vi "05. Native MQTT Delegation.vi"() -> ()   [LabVIEW 2019]
uses:
  Actor/Request -- cluster.ctl
  <vilib>/LabVIEW Open Source Project/MQTT Control Packets/Control Packets/ControlPacket/ControlPacket.lvclass/ControlPacket.ctl
  d83398bf-d288-4447-9c56-1851baa950d7.vi
  <vilib>/LabVIEW Open Source Project/MQTT Control Packets/Control Packets/PUBLISH/PUBLISH.lvclass
  C:/Program Files (x86)/National Instruments/LabVIEW 2019/vi.lib/LabVIEW Open Source Project/MQTT Control Packets/Control Packets/ControlPacket/ControlPacket.lvclass
  <vilib>/JDP Science/JSONtext/JSON text to Variant.vi
  <vilib>/Utility/error.llb/Error Cluster From Error Code.vi
  <vilib>/JDP Science/JSONtext/LVClass Serializer/JSONtext LVClass Serializer.lvclass
  <vilib>/ErrorRing/Error Ring.xnode
  <vilib>/LabVIEW Open Source Project/MQTT Control Packets/Control Packets/ControlPacket/ControlPacket.lvclass
  <vilib>/JDP Science/JSONtext/JSONtext.lvlib
  <vilib>/ptbypt/NI_PtbyPt.lvlib
panel:
  in  "amplitude":dbl(slide)=2.0 scale=0.0..10.0
  out "<JSON>Response":string
  out "<JSON>":string caption="<JSON>Request"
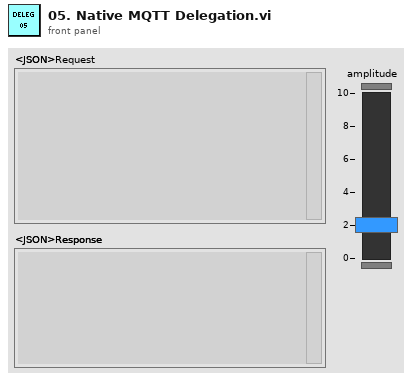
[diagram p1: front panel]
types:
  T1 = typedef "Actor Private Data.ctl" = cluster{"Client":refnum<class "Client.lvclass">, "QualifiedName":string, "EventReg":refnum<event-registration>, "Private Events":T2}
  T2 = typedef "Actor Private Events -- cluster.ctl" = cluster{"Stop":refnum<user-event>, "Subscribe":refnum<user-event>, "Unsubscribe":refnum<user-event>, "publish":refnum<user-event>}
  T3 = typedef "Request -- cluster.ctl" = cluster{"method":string, "<JSON>params":string, "id":string, "reply-topic":string}
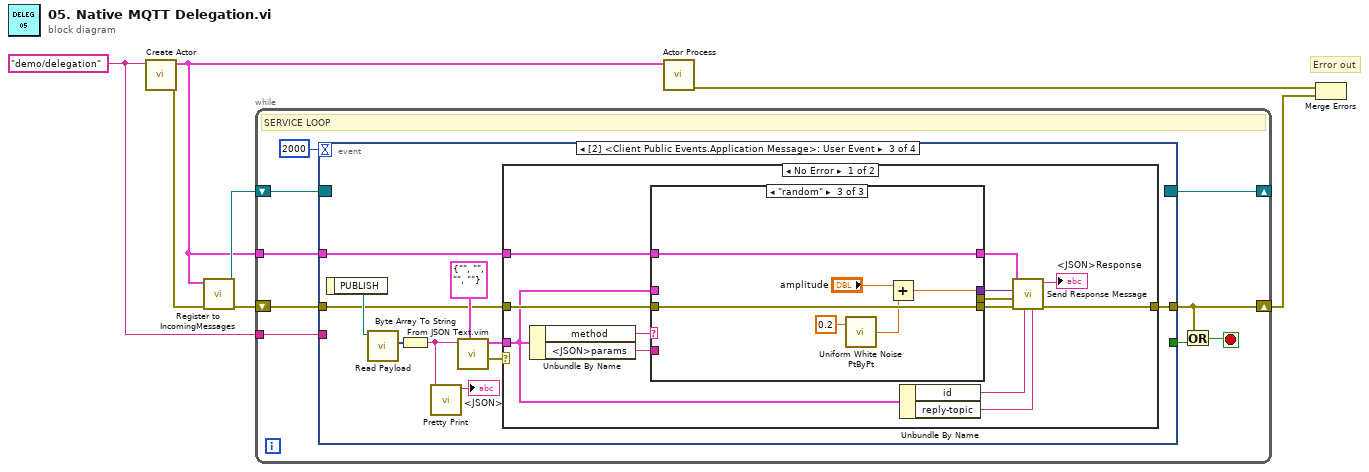
[diagram p0: block diagram]
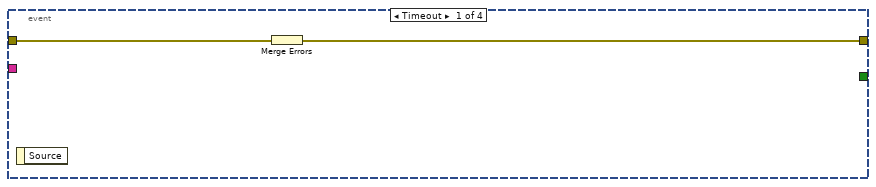
[diagram p2: hidden frame]
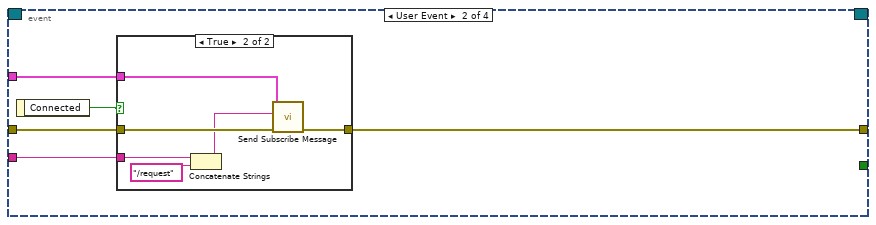
[diagram p3: hidden frame]
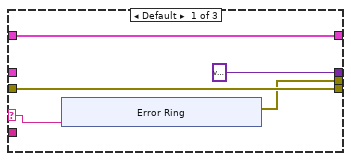
[diagram p5: hidden frame]
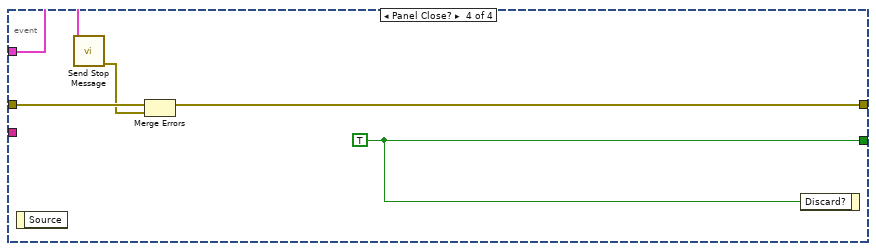
[diagram p8: hidden frame]
diagram:
  w2 = "demo/delegation" ("QualifiedName")
  # "Error out"
  n1 = call "Create Actor.vi"("QualifiedName"=w2) -> ("error out"=w6:errorcluster, "Actor Class"=w4:T1)  [unwired: 9 in]
  n2 = call "Register to IncomingMessages.vi"("error in"=w6, "Actor Class"=w4) -> ("error out"=w3:errorcluster, "Incoming Messages"=w5:refnum<event-registration>)  [unwired: 8 in]
  n3 = while {
    tunnel: w4 -> [w14]
    shift-right: [w11] -> _
    shift-left: w5 -> [w12]
    shift-right: [w9] -> w1
    shift-left: w3 -> [w10]
    tunnel: w2 -> [w8]
    stop <- w15 stop-if-true
    # "SERVICE LOOP"
    n4 = event shown="[2] <Client Public Events.Application Message>: User Event" {
      selector: w12 -> [_ _ _ _]
      dyn-events: [_ _ _ _] -> w11
      timeout: 2000 -> [_ _ _ _]
      tunnel: [_ _ _ w80] -> w16
      tunnel: w14 -> [_ w21 w35 w79]
      tunnel: [w17 w22 w33 w76] -> w9
      tunnel: w10 -> [w18 w23 w34 w78]
      tunnel: w8 -> [_ w19 _ _]
      event Timeout {
        n5 = event-data() -> ()  [unwired: 1 in, 1 out]
        n6 = Merge Errors(w18) -> (w17:errorcluster)
      }
      event User Event {
        n7 = event-data() -> ("Connected"=w20:bool)  [unwired: 1 in]
        n8 = case shown="True" w20 {
          tunnel: w23 -> [w24 w30]
          tunnel: [w24 w29] -> w22
          tunnel: w21 -> [_ w28]
          tunnel: w19 -> [_ w27]
          frame False {
          }
          frame True {
            n9 = Concatenate Strings(w27, "/request" ("QualifiedName")) -> (w25:string)
            n10 = call "Send Subscribe Message.vi"("error in"=w30, "Topic"=w25, "Actor Class"=w28) -> ("error out"=w29:errorcluster)  [unwired: 8 in]
          }
        }
      }
      event User Event {
        n11 = event-data() -> ("PUBLISH"=w40:refnum<class "PUBLISH.lvclass">)  [unwired: 1 in]
        n12 = call <vilib>:"Read Payload.vi"("ControlPacket in"=w40) -> ("Payload"=w39:u8[])  [unwired: 9 in, 1 out]
        n13 = Byte Array To String(unsigned byte array=w39) -> (string=w32:string)
        n14 = call <vilib>:"Pretty Print.vi"("JSON"=w32) -> ("<JSON>"=→"<JSON>":string)  [unwired: 8 in, 2 out]
        n15 = call "From JSON Text.vim"("Data Type and Default Value"=T3 {"method"="", "<JSON>params"="", "id"="", "reply-topic"=""} ("request"), "JSON"=w32) -> ("error out"=w37:errorcluster, "Data out"=w36:T3)  [unwired: 8 in]
        n16 = case shown="No Error" w37 {
          tunnel: w36 -> [w42 _]
          tunnel: w35 -> [w51 _]
          tunnel: w34 -> [w50 w75]
          tunnel: [w48 w75] -> w33
          frame No Error {
            n17 = Unbundle By Name(w42) -> ("method"=w53:string, "<JSON>params"=w52:string)
            n18 = case shown="\"random\"" w53 {
              selector: w53 -> [w54 _ _]
              tunnel: w52 -> [_ _ _]
              tunnel: w51 -> [w57 w67 w73]
              tunnel: w50 -> [w58 w68 w74]
              tunnel: [w58 w68 w74] -> w47
              tunnel: [w57 w67 w73] -> w49
              tunnel: [w56 _ _] -> w44
              tunnel: [variant ("result") w66 w69] -> w43
              tunnel: w42 -> [_ w66 _]
              frame Default {
                n19 = xnode "Error Ring"("parameter 0"=w54) -> ("error out"=w56:errorcluster)
              }
              frame "echo" {
              }
              frame "random" {
                n20 = call <vilib>:"Uniform White Noise PtByPt.vi"("amplitude"=0.2) -> ("uniform white noise"=w72:dbl)  [unwired: 2 in]
                n21 = Add(x="amplitude", y=w72) -> (x+y=w69:dbl)
              }
            }
            n22 = Unbundle By Name(w42) -> ("id"=w46:string, "reply-topic"=w45:string)
            n23 = call "Send Response Message.vi"("topic"=w45, "id"=w46, "error in"=w47, "request error"=w44, "result"=w43, "Actor Class"=w49) -> ("error out"=w48:errorcluster, "<JSON>Response"=→"<JSON>Response":string)  [unwired: 4 in]
          }
          frame Error {
            # "Invalid request payload"
          }
        }
      }
      event Panel Close? {
        w80 = TRUE ("Discard?")
        n24 = event-data() -> ()  [unwired: 1 in, 1 out]
        n25 = call "Send Stop Message.vi"("Actor Class"=w79) -> ("error out"=w77:errorcluster)  [unwired: 10 in]
        n26 = Merge Errors(w78, w77) -> (w76:errorcluster)
        n27 = event-data("Discard?"=w80) -> ()  [unwired: 1 in, 1 out]
      }
    }
    n28 = Or(x=w9, y=w16) -> (x .or. y?=w15:bool)
  }
  n29 = call "Actor Process.vi"("Actor Class"=w4) -> ("error out"=w7:errorcluster)  [unwired: 10 in]
  n30 = Merge Errors(w7, w1) -> ()  [unwired: 1 out]
